vi "Bangbang Shooter Control.vi"(6 "Loop Interval":dbl, 7 "IIR Filter Power":dbl, 8 "Target RPM":dbl, 10 "Current RPM":dbl, 11 "MotorDevRef":T1={"DeviceStatus"={"status"=FALSE, "code"=0, "source"=""}, "Type"=enum."PWM", "PWM"={"Digital Module"=enum."Digital Module 1", "PWM Channel"=enum."Invalid", "DeadBand"={"Name"="", "maxPositivePwm"=0, "minPositivePwm"=0, "centerPwm"=0, "maxNegativePwm"=0, "minNegativePwm"=0, "angularRange"=0}}, "CAN"={"Device Number"=0, "Control Mode"=enum."Percent VBus", "Semaphore"=refnum, "Max Vout"=12.0}, "Invert"=FALSE, "TransformRef"=refnum, "InvTransformRef"=refnum}) -> (2 "Motor Output":dbl)   [LabVIEW 2013]
uses:
  <vilib>/Rock Robotics/WPI/MotorControl/WPI_MotorControlDeviceRef.ctl
  <vilib>/Rock Robotics/SystemInterfaces/Typedef/FPGA_TypedefDigitalModule.ctl
  <vilib>/Rock Robotics/SystemInterfaces/DIO/FPGA_DIOPWMChannel.ctl
  <vilib>/Rock Robotics/WPI/PWM/WPI_PWMDeadband.ctl
  <vilib>/Rock Robotics/WPI/CAN/Jaguar/SubVIs/WPI_CANJaguar_ControlMode.ctl
  <vilib>/Rock Robotics/WPI/PWM/WPI_PWMTransform_ConPane.ctl
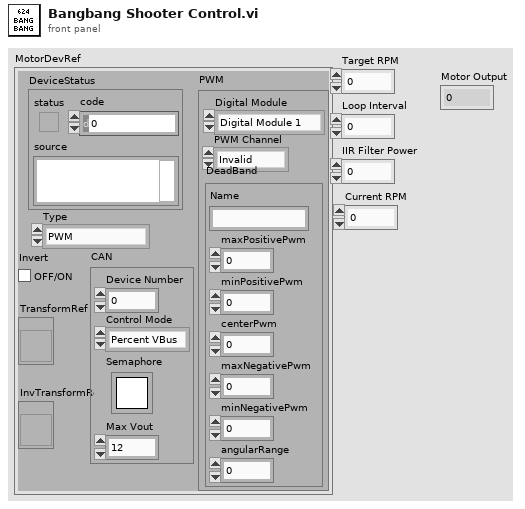
[diagram p1: front panel]
types:
  T1 = typedef "WPI_MotorControlDeviceRef.ctl" = cluster{"DeviceStatus":errorcluster, "Type":enum16{"PWM", "CAN"}, "PWM":cluster{"Digital Module":T2, "PWM Channel":T3, "DeadBand":T4}, "CAN":cluster{"Device Number":u8, "Control Mode":T5, "Semaphore":T6, "Max Vout":dbl}, "Invert":bool, "TransformRef":T7, "InvTransformRef":T7}
  T2 = typedef "FPGA_TypedefDigitalModule.ctl" = enum16{"Digital Module 1", "Digital Module 2"}
  T3 = typedef "FPGA_DIOPWMChannel.ctl" = enum8{"PWM 1", "PWM 2", "PWM 3", "PWM 4", "PWM 5", "PWM 6", "PWM 7", "PWM 8", "PWM 9", "PWM 10", "Invalid"}
  T4 = typedef "WPI_PWMDeadband.ctl" = cluster{"Name":string, "maxPositivePwm":i32, "minPositivePwm":i32, "centerPwm":i32, "maxNegativePwm":i32, "minNegativePwm":i32, "angularRange":u16}
  T5 = typedef "WPI_CANJaguar_ControlMode.ctl" = enum8{"Percent VBus", "Current", "Speed", "Position", "Voltage"}
  T6 = typedef "Semaphore RefNum" = refnum<k1>
  T7 = typedef "WPI_PWMTransform_ConPane.ctl" = refnum<vi>
  T8 = typedef "WPI_CounterDevRef.ctl" = cluster{"DevStatus":errorcluster, "CntIndex":T9}
  T9 = typedef "FPGA_CounterCtrSystemIndex.ctl" = enum8{"Ctr 0", "Ctr 1", "Ctr 2", "Ctr 3", "Ctr 4", "Ctr 5", "Ctr 6", "Ctr 7", "Invalid"}
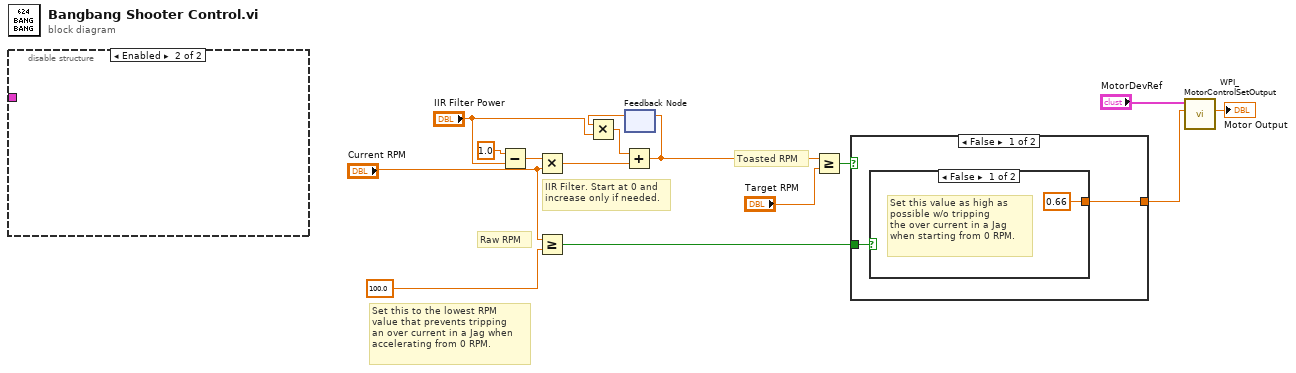
[diagram p0: block diagram]
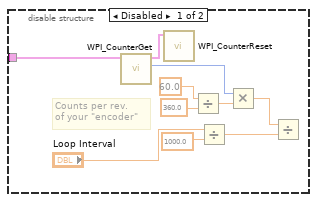
[diagram p2: hidden frame]
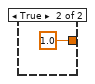
[diagram p3: hidden frame]
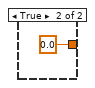
[diagram p4: hidden frame]
diagram:
  # "Toasted RPM"
  # "Raw RPM"
  # "Set this to the lowest RPM \nvalue that prevents tripping\nan over current in a Jag when \naccelerating from 0 RPM."
  # "IIR Filter. Start at 0 and \nincrease only if needed."
  n1 = disable-structure shown="Enabled" {
    disable-tunnel: _ -> [w16 _]
    frame Disabled {
      # "Counts per rev. \nof your \"encoder\""
      n2 = call <vilib>:"WPI_CounterGet.vi"("CounterDevRef in"=w16) -> ("Value"=w21:i32, "CounterDevRef out"=w25:T8)  [unwired: 5 in, 4 out]
      n3 = call <vilib>:"WPI_CounterReset.vi"("CounterDevRef in"=w25) -> ()  [unwired: 9 in, 2 out]
      n4 = Divide(x=60.0, y=360.0) -> (x/y=w22:dbl)
      n5 = Divide(x="Loop Interval", y=1000.0) -> (x/y=w19:dbl)
      n6 = Multiply(x=w21, y=w22) -> (x*y=w20:dbl)
      n7 = Divide(x=w20, y=w19) -> ()  [unwired: 1 out]
    }
    frame Enabled {
    }
  }
  n8 = Subtract(x=1.0, y="IIR Filter Power") -> (x-y=w9:dbl)
  n9 = Multiply(x=w9, y="Current RPM") -> (x*y=w13:dbl)
  n10 = Greater Or Equal?(x="Current RPM", y=100.0) -> (x >= y?=w5:bool)
  n11 = feedback #1() -> (w14:dbl)  [unwired: 1 in]
  n12 = Multiply(x=w14, y="IIR Filter Power") -> (x*y=w12:dbl)
  n13 = Add(x=w12, y=w13) -> (x+y=w10:dbl)
  n14 = feedback-in #1(w10) -> ()
  n15 = Greater Or Equal?(x=w10, y="Target RPM") -> (x >= y?=w7:bool)
  n16 = case shown="False" w7 {
    tunnel: [w26 0.0] -> w6
    tunnel: w5 -> [w27 _]
    frame False {
      n17 = case shown="False" w27 {
        tunnel: [0.66 1.0] -> w26
        frame False {
          # "Set this value as high as \npossible w/o tripping\nthe over current in a Jag\nwhen starting from 0 RPM."
        }
        frame True {
        }
      }
    }
    frame True {
    }
  }
  n18 = call <vilib>:"WPI_MotorControlSetOutput.vi"("Output"=w6, "MotorControlDevRef"="MotorDevRef") -> ("Motor Output"=→"Motor Output":dbl)  [unwired: 7 in, 2 out]
